vi "GetTopLevelPath.vi"(8 "error in":errorcluster) -> (0 "error out":errorcluster, 3 "path":path)   [LabVIEW 2010]
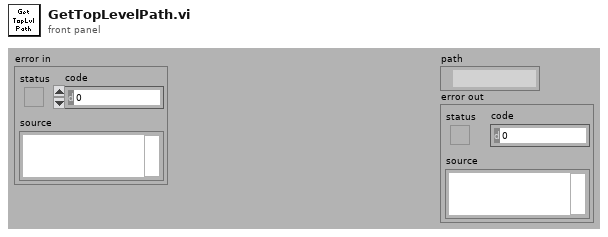
[diagram p1: front panel]
types:
  T1 = enum32{"invalid app kind", "Development System", "Run Time System", "Student Edition", "Embedded LabVIEW", "Evaluation", "Custom"}
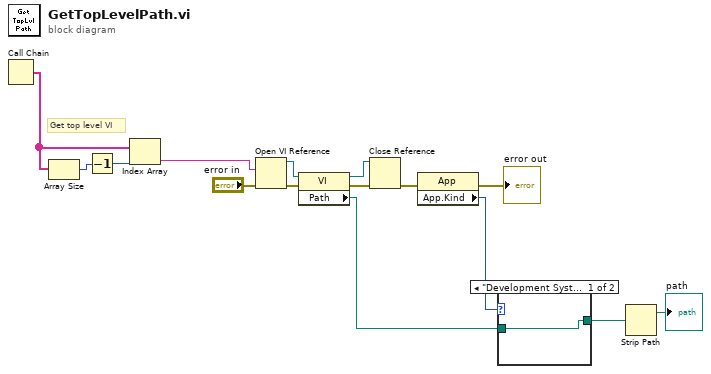
[diagram p0: block diagram]
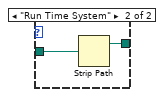
[diagram p2: hidden frame]
diagram:
  # "Get top level VI"
  n1 = Call Chain() -> (call chain=w9:string[])
  n2 = Array Size(array=w9) -> (size(s)=w12:i32)
  n3 = Decrement(x=w12) -> (x-1=w11:i32)
  n4 = Index Array(array=w9, index=w11) -> (element=w10:string)
  n5 = Open VI Reference(vi path=w10, error in (no error)="error in") -> (vi reference=w13:refnum<vi>, error out=w14:errorcluster)  [unwired: 4 in]
  n6 = property class="VI"(reference=w13, error in=w14) -> (reference out=w1:refnum<vi>, error out=w4:errorcluster, "Path"=w8:path)
  n7 = Close Reference(reference=w1, error in (no error)=w4) -> (error out=w3:errorcluster)
  n8 = property class="App"(error in=w3) -> (error out=→"error out":errorcluster, "App.Kind"=w7:T1)  [unwired: 1 in, 1 out]
  n9 = case shown="\"Development System\", Default" w7 {
    tunnel: w8 -> [w16 w18]
    tunnel: [w16 w17] -> w6
    frame "Development System", Default {
    }
    frame "Run Time System" {
      n10 = Strip Path(path=w18) -> (stripped path=w17:path)  [unwired: 1 out]
    }
  }
  n11 = Strip Path(path=w6) -> (stripped path=→"path":path)  [unwired: 1 out]
